vi "Read SCB via ESP (SubVI).vi"(0 "COM Port Input":refnum<visa-resource-name>, 2 "Manual Write Command":bool, 3 "Write/Read Wait (ms)":u32=10, 4 "Timeout (ms)":u32=10, 5 "Tare":bool) -> (14 "Weight (Grams)":dbl, 15 "COM Output":T2, 16 "SCB Output":T1, 19 "Error Output":errorcluster)   [LabVIEW 2011]
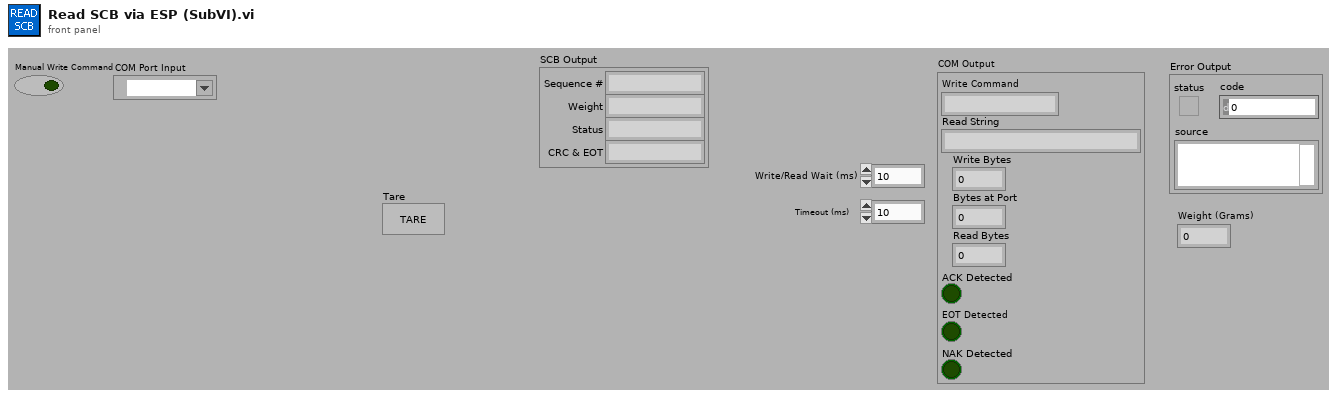
[diagram p1: front panel]
types:
  T1 = cluster{"Sequence #":string, "Weight":string, "Status":string, "CRC & EOT":string}
  T2 = cluster{"Write Command":string, "Read String":string, "Write Bytes":u32, "Bytes at Port":u32, "Read Bytes":u32, "ACK Detected":bool, "EOT Detected":bool, "NAK Detected":bool}
  T3 = cluster{"[0]":string, "[1]":string, "[2]":string, "[3]":string}
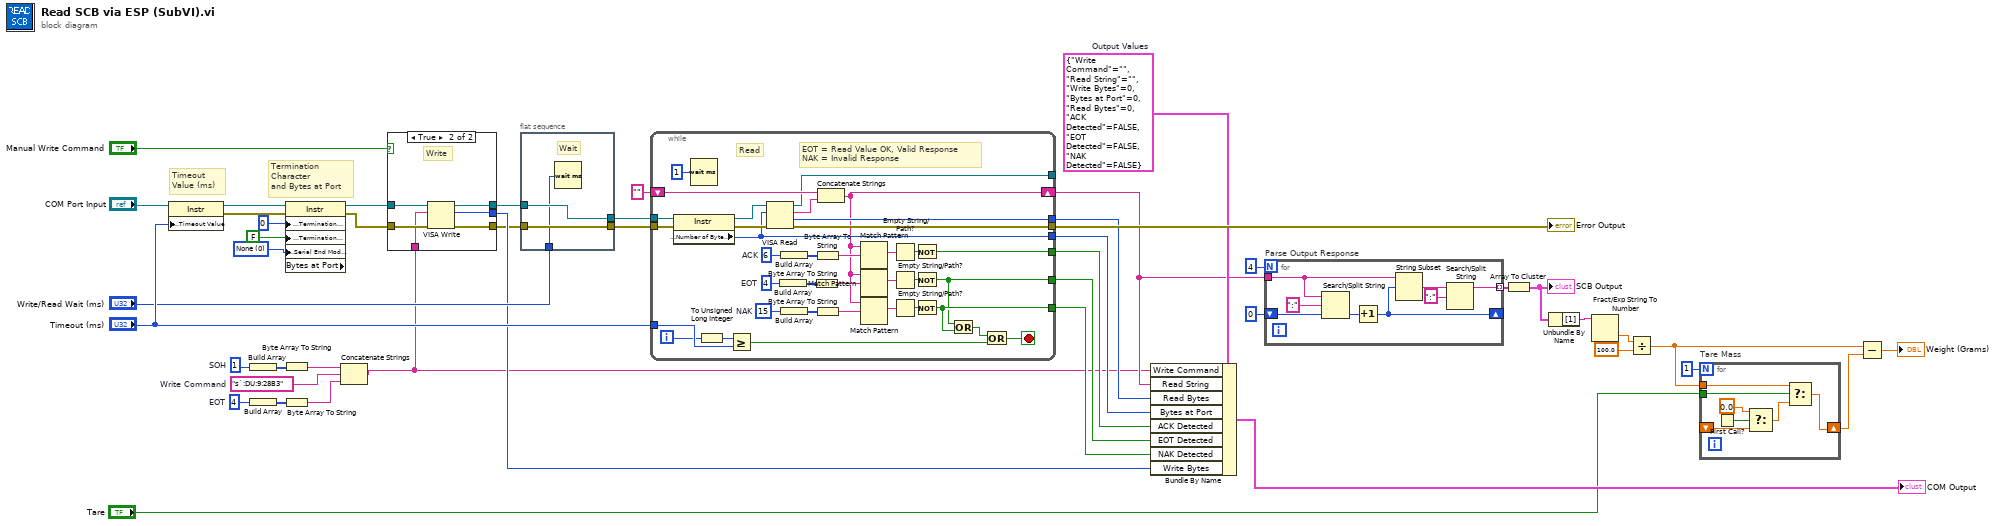
[diagram p0: block diagram]
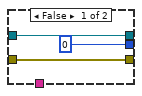
[diagram p2: hidden frame]
diagram:
  w12 = u8 4  # EOT
  w10 = u8 1  # SOH
  w8 = "s`:DU:9:28B3"  # Write Command
  w39 = T2 {"Write Command"="", "Read String"="", "Write Bytes"=0, "Bytes at Port"=0, "Read Bytes"=0, "ACK Detected"=FALSE, "EOT Detected"=FALSE, "NAK Detected"=FALSE}  # Output Values
  w30 = u16 0 items=["None", "LastBit", "TermChar"] ("ASRLEndIn")
  # "Timeout \nValue (ms)"
  # "Termination \nCharacter\nand Bytes at Port"
  n1 = property class="Instr"(reference="COM Port Input", "General Settings:Timeout Value"="Timeout (ms)") -> (reference out=w34:refnum<visa-resource-name>, error out=w33:errorcluster)  [unwired: 1 in]
  n2 = Build Array(w10) -> (w11:u8[])
  n3 = Build Array(w12) -> (w13:u8[])
  n4 = Byte Array To String(unsigned byte array=w11) -> (string=w9:string)
  n5 = Byte Array To String(unsigned byte array=w13) -> (string=w7:string)
  n6 = property class="Instr" props=["Message Based Settings:Termination Character", "Message Based Settings:Termination Character Enable", "Serial Settings:Serial End Mode for Reads", "Bytes at Port"](reference=w34, error in=w33, "Message Based Settings:Termination Character"=u8 0 ("Termination Char"), "Message Based Settings:Termination Character Enable"=FALSE ("enable"), "Serial Settings:Serial End Mode for Reads"=w30) -> (reference out=w24:refnum<visa-resource-name>, error out=w23:errorcluster)  [unwired: 1 out]
  n7 = Concatenate Strings(w9, w8, w7) -> (w6:string)
  n8 = case shown="True" "Manual Write Command" {
    tunnel: [w49 w55] -> w37
    tunnel: w24 -> [w49 w54]
    tunnel: w23 -> [w48 w53]
    tunnel: [w48 w52] -> w35
    tunnel: [u32 0 ("return count") w51] -> w40
    tunnel: w6 -> [_ w50]
    frame False {
    }
    frame True {
      # "Write"
      n9 = VISA Write(VISA resource name=w54, write buffer=w50, error in (no error)=w53) -> (VISA resource name out=w55:refnum<visa-resource-name>, return count=w51:u32, error out=w52:errorcluster)
    }
  }
  n10 = flat-sequence {
    tunnel: w35 -> [w58]
    tunnel: [w58] -> w36
    tunnel: w37 -> [w57]
    tunnel: [w57] -> w38
    tunnel: "Write/Read Wait (ms)" -> [w56]
    frame #0 {
      # "Wait"
      n11 = Wait (ms)(milliseconds to wait=w56) -> ()  [unwired: 1 out]
    }
  }
  n12 = while {
    shift-left: "" -> [w93]
    shift-right: [w68] -> w22
    tunnel: [w91] -> w41
    tunnel: w36 -> [w84]
    tunnel: w38 -> [w83]
    tunnel: [w90] -> _
    tunnel: [w89] -> w18
    tunnel: [w81] -> w26
    tunnel: [w80] -> w28
    tunnel: [w64] -> w27
    tunnel: [w63] -> w29
    tunnel: "Timeout (ms)" -> [w62]
    i -> [w59]
    stop <- w67 stop-if-true
    w70 = u8 15  # NAK
    w76 = u8 4  # EOT
    w86 = u8 6  # ACK
    # "EOT = Read Value OK, Valid Response\nNAK = Invalid Response"
    # "Read"
    n13 = property class="Instr"(reference=w83, error in=w84) -> (reference out=w82:refnum<visa-resource-name>, error out=w94:errorcluster, "Serial Settings:Number of Bytes at Serial Port"=w81:u32)
    n14 = Wait (ms)(milliseconds to wait=u32 1) -> ()  [unwired: 1 out]
    n15 = To Unsigned Long Integer(number=w59) -> (unsigned 32bit integer=w60:u32)
    n16 = Greater Or Equal?(x=w60, y=w62) -> (x >= y?=w66:bool)
    n17 = VISA Read(VISA resource name=w82, byte count=w81, error in (no error)=w94) -> (VISA resource name out=w90:refnum<visa-resource-name>, read buffer=w92:string, return count=w89:u32, error out=w91:errorcluster)
    n18 = Build Array(w76) -> (w75:u8[])
    n19 = Build Array(w86) -> (w85:u8[])
    n20 = Build Array(w70) -> (w69:u8[])
    n21 = Byte Array To String(unsigned byte array=w75) -> (string=w77:string)
    n22 = Byte Array To String(unsigned byte array=w85) -> (string=w74:string)
    n23 = Byte Array To String(unsigned byte array=w69) -> (string=w71:string)
    n24 = Concatenate Strings(w93, w92) -> (w68:string)
    n25 = Match Pattern(string=w68, regular expression=w74) -> (match substring=w87:string)  [unwired: 4 out]
    n26 = Match Pattern(string=w68, regular expression=w77) -> (match substring=w78:string)  [unwired: 4 out]
    n27 = Match Pattern(string=w68, regular expression=w71) -> (match substring=w73:string)  [unwired: 4 out]
    n28 = Empty String/Path?(string/path=w87) -> (empty?=w88:bool)
    n29 = Empty String/Path?(string/path=w78) -> (empty?=w79:bool)
    n30 = Empty String/Path?(string/path=w73) -> (empty?=w72:bool)
    n31 = Not(x=w88) -> (.not. x?=w80:bool)
    n32 = Not(x=w79) -> (.not. x?=w63:bool)
    n33 = Not(x=w72) -> (.not. x?=w64:bool)
    n34 = Or(x=w63, y=w64) -> (x .or. y?=w65:bool)
    n35 = Or(x=w65, y=w66) -> (x .or. y?=w67:bool)
  }
  "Error Output" <- w41
  n36 = Bundle By Name(cluster=w39, "Write Command"=w6, "Read String"=w22, "Read Bytes"=w18, "Bytes at Port"=w26, "ACK Detected"=w28, "EOT Detected"=w29, "NAK Detected"=w27, "Write Bytes"=w40) -> (→"COM Output":T2)
  n37 = for "Parse Output Response" {
    N: 4 ("Numeric") -> [_]
    shift-right: [w99] -> _
    shift-left: 0 ("offset of match") -> [w100]
    tunnel: w22 -> [w98]
    tunnel: [w95] -> w19 mode=indexing
    n38 = Search/Split String(string=w98, search string/char (-)=":", offset (0)=w100) -> (offset of match=w101:i32)  [unwired: 2 out]
    n39 = Increment(x=w101) -> (x+1=w99:i32)
    n40 = String Subset(string=w98, offset (0)=w99) -> (substring=w96:string)  [unwired: 1 out]
    n41 = Search/Split String(string=w96, search string/char (-)=":") -> (substring before match=w95:string)  [unwired: 3 out]
  }
  n42 = Array To Cluster(array=w19) -> (cluster=w14:T3)
  "SCB Output" <- w14
  n43 = Unbundle By Name(w14) -> ("[1]"=w15:string)
  n44 = Fract/Exp String To Number(string=w15) -> (number=w16:dbl)  [unwired: 4 out]
  n45 = Divide(x=w16, y=100.0) -> (x/y=w1:dbl)
  n46 = for "Tare Mass" {
    N: 1 -> [_]
    tunnel: w1 -> [w109]
    shift-right: [w108] -> w4
    shift-left: _ -> [w105]
    tunnel: "Tare" -> [w103]
    n47 = First Call?() -> (First Call?: T/F=w106:bool)
    n48 = Select(t=0.0, s=w106, f=w105) -> (s? t:f=w104:dbl)
    n49 = Select(t=w109, s=w103, f=w104) -> (s? t:f=w108:dbl)
  }
  n50 = Subtract(x=w1, y=w4) -> (x-y=→"Weight (Grams)":dbl)
